vi "Combine MofI.vi"(8 "Rotational Mass 4":T1={"Ratio (out/in)"=1.0, "Moment of Inertia (kg m^2)"=0.0} {"Moment of Inertia (kg m^2)" format="%#_3p"}, 9 "Rotational Mass 3":T1={"Ratio (out/in)"=1.0, "Moment of Inertia (kg m^2)"=0.0} {"Moment of Inertia (kg m^2)" format="%#_3p"}, 10 "Rotational Mass 2":T1={"Ratio (out/in)"=1.0, "Moment of Inertia (kg m^2)"=0.0} {"Moment of Inertia (kg m^2)" format="%#_3p"}, 11 "Rotational Mass 1":T1={"Ratio (out/in)"=1.0, "Moment of Inertia (kg m^2)"=0.0} {"Moment of Inertia (kg m^2)" format="%#_3p"}) -> (3 "Combined":T1 {"Moment of Inertia (kg m^2)" format="%#_3p"})   [LabVIEW 2019]
uses:
  Motor Physical Values.ctl
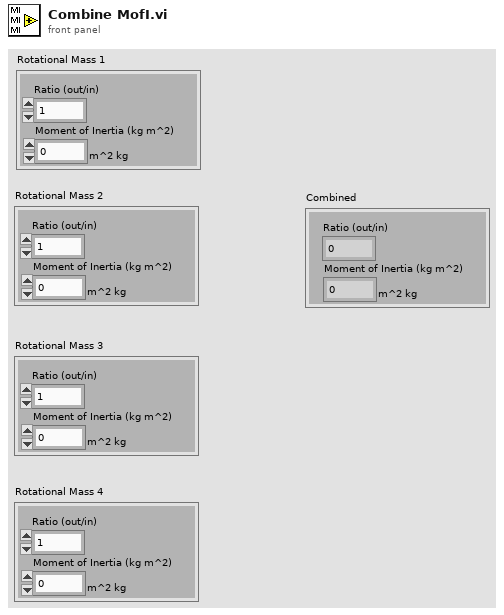
[diagram p1: front panel]
types:
  T1 = typedef "Motor Physical Values.ctl" = cluster{"Ratio (out/in)":dbl, "Moment of Inertia (kg m^2)":dbl[unit]}
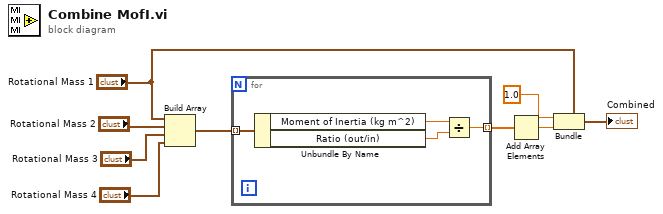
[diagram p0: block diagram]
diagram:
  n1 = Build Array("Rotational Mass 1", "Rotational Mass 2", "Rotational Mass 3", "Rotational Mass 4") -> (w6:T1[])
  n2 = for {
    tunnel: w6 -> [w13] mode=indexing
    tunnel: [w10] -> w5 mode=indexing
    n3 = Unbundle By Name(w13) -> ("Moment of Inertia (kg m^2)"=w12:dbl[unit], "Ratio (out/in)"=w11:dbl)
    n4 = Divide(x=w12, y=w11) -> (x/y=w10:dbl[unit])
  }
  n5 = Add Array Elements(numeric array=w5) -> (sum=w4:dbl[unit])
  n6 = Bundle(cluster="Rotational Mass 1", "Ratio (out/in)"=1.0, "Moment of Inertia (kg m^2)"=w4) -> (→"Combined":T1)
